vi "Set Body.vi"(8 "error in (no error)":errorcluster, 10 "Body":string, 11 "Response in":refnum<class "Response.lvclass">) -> (0 "error out":errorcluster, 3 "Response out":refnum<class "Response.lvclass">)   [LabVIEW 2023, in "Response.lvclass"]
uses:
  Response.lvclass
  Response.lvclass/Response.ctl
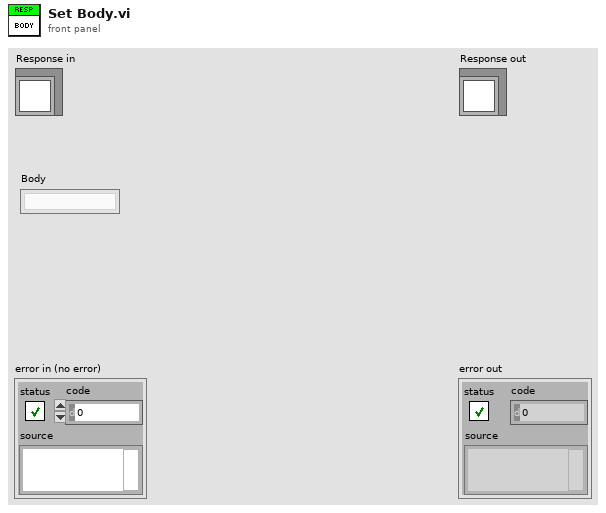
[diagram p1: front panel]
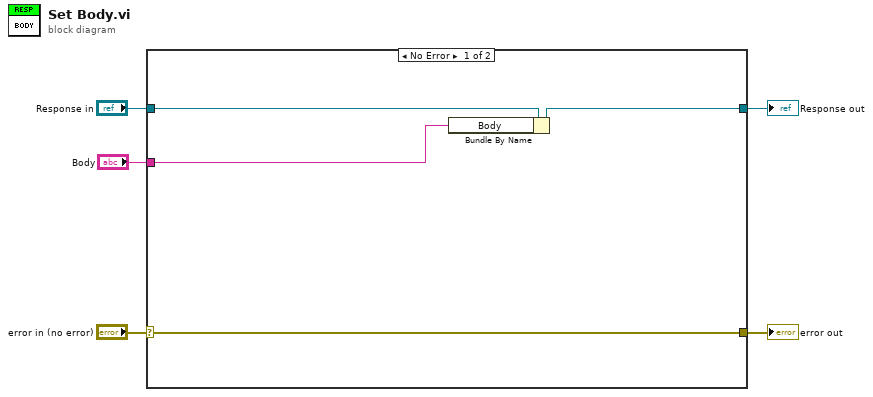
[diagram p0: block diagram]
diagram:
  n1 = case shown="No Error" "error in (no error)" {
    selector: "error in (no error)" -> [w9 w11]
    tunnel: [w9 w11] -> w4
    tunnel: [w7 w10] -> w2
    tunnel: "Response in" -> [w8 w10]
    tunnel: "Body" -> [w6 _]
    frame No Error {
      n2 = Bundle By Name(cluster=w8, "Body"=w6) -> (w7:refnum<class "Response.lvclass">)
    }
    frame Error {
    }
  }
  "error out" <- w4
  "Response out" <- w2
